vi "Lab Panel V5.24.2.vi"() -> ()   [LabVIEW 2013] (continued)
                          frame False {
                          }
                          frame True {
                            n2517 = Bundle(cluster=w4678, "amps"=w4682, "volts"=w4681, "pf"=w4680) -> (w4679:cluster{"amps":dbl, "volts":dbl, "pf":dbl})
                            n2518 = local write "ON L05-2"(w4679) -> ()
                          }
                        }
                      }
                      frame #1 {
                        n2519 = Unbundle(w4687) -> ("amps"=w4686:dbl, "volts"=w4685:dbl, "pf"=w4684:dbl)
                        n2520 = case shown="True" w4688 {
                          tunnel: w4695 -> [_ w4727]
                          tunnel: w4694 -> [_ w4734]
                          tunnel: w4693 -> [_ _]
                          tunnel: w4692 -> [_ _]
                          tunnel: w4691 -> [_ w4733]
                          tunnel: w4690 -> [_ w4732]
                          tunnel: w4689 -> [_ w4697]
                          tunnel: w4686 -> [_ w4729]
                          tunnel: w4685 -> [_ w4728]
                          tunnel: w4684 -> [_ w4726]
                          tunnel: w4683 -> [_ w4718]
                          frame False {
                          }
                          frame True {
                            n2521 = local read "TDMS LAB05-2"() -> (w4731:refnum<k34>)
                            n2522 = Build Array(w4728) -> (w4723:dbl[])
                            n2523 = Build Array(w4726) -> (w4722:dbl[])
                            n2524 = Build Array(w4733) -> (w4721:dbl[])
                            n2525 = Build Array(w4734) -> (w4720:dbl[])
                            n2526 = Build Array(w4729) -> (w4725:dbl[])
                            n2527 = Build Array(w4727) -> (w4724:dbl[])
                            n2528 = Build Array(w4732) -> (w4719:dbl[])
                            n2529 = Build Array("AMPS ON", "AMPS OFF", "VOLTS", "PF", "TEMP Live", "TEMP Neut", "CYCLE") -> (w4702:string[])
                            n2530 = Bundle By Name("Y"=w4725, "t0"=w4718) -> (w4717:waveform(dbl))  [unwired: 1 in]
                            n2531 = Bundle By Name("Y"=w4724, "t0"=w4718) -> (w4716:waveform(dbl))  [unwired: 1 in]
                            n2532 = Bundle By Name("Y"=w4723, "t0"=w4718) -> (w4715:waveform(dbl))  [unwired: 1 in]
                            n2533 = Bundle By Name("Y"=w4722, "t0"=w4718) -> (w4714:waveform(dbl))  [unwired: 1 in]
                            n2534 = Bundle By Name("Y"=w4721, "t0"=w4718) -> (w4713:waveform(dbl))  [unwired: 1 in]
                            n2535 = Bundle By Name("Y"=w4720, "t0"=w4718) -> (w4712:waveform(dbl))  [unwired: 1 in]
                            n2536 = Bundle By Name("Y"=w4719, "t0"=w4718) -> (w4711:waveform(dbl))  [unwired: 1 in]
                            n2537 = Build Array(w4717, w4716, w4715, w4714, w4713, w4712, w4711) -> (w4710:waveform(dbl)[])
                            n2538 = TDMS Write(0:w4731, 5:"TEST VALUES", 7:w4702, 9:w4710) -> (4:w4701:refnum<k34>, 6:w4700:string, 15:w4699:errorcluster)  [unwired: 2 in, 1 out]
                            n2539 = TDMS Write(0:w4701, 5:w4700, 7:"TIME", 9:w4697, 11:w4699) -> (15:w4696:errorcluster)  [unwired: 1 in, 3 out]
                            n2540 = local write "data file error"(w4696) -> ()
                          }
                        }
                      }
                    }
                  }
                }
              }
            }
          }
          frame #14 {
            # "display test values on chart"
            n2541 = local read "jig cycle"() -> (w4739:dbl)
            n2542 = local read "on loops"() -> (w4741:dbl)
            n2543 = Add(x=w4741, y=2) -> (x+y=w4738:dbl)
            n2544 = Equal?(x=w4739, y=1) -> (x = y?=w4737:bool)
            n2545 = Equal?(x=w4739, y=w4738) -> (x = y?=w4736:bool)
            n2546 = Or(x=w4737, y=w4736) -> (x .or. y?=w4735:bool)
            "graph flag" <- w4735
            n2547 = global write "Global display 3.vi" "graph flag"(w4735) -> ()
            n2548 = case shown="True" w4735 {
              frame False {
              }
              frame True {
                n2549 = local read "SIG LAB05-1"() -> (w4784:T2)
                n2550 = local read "SIG LAB04-2"() -> (w4785:T2)
                n2551 = local read "SIG LAB05-2"() -> (w4783:T2)
                n2552 = local read "SIG LAB04-1"() -> (w4786:T2)
                n2553 = local read "SIG LAB03-1"() -> (w4788:T2)
                n2554 = local read "SIG LAB03-2"() -> (w4787:T2)
                n2555 = local read "SIG LAB01-1"() -> (w4792:T2)
                n2556 = local read "SIG LAB02-2"() -> (w4789:T2)
                n2557 = local read "SIG LAB02-1"() -> (w4790:T2)
                n2558 = local read "SIG LAB01-2"() -> (w4791:T2)
                n2559 = Unbundle(w4785) -> ("AMPS"=w4775:dbl, "VOLTS"=w4765:dbl, "Tmp Live"=w4755:dbl, "Tmp Neut"=w4745:dbl)  [unwired: 1 out]
                n2560 = Unbundle(w4784) -> ("AMPS"=w4774:dbl, "VOLTS"=w4764:dbl, "Tmp Live"=w4754:dbl, "Tmp Neut"=w4744:dbl)  [unwired: 1 out]
                n2561 = Unbundle(w4783) -> ("AMPS"=w4773:dbl, "VOLTS"=w4763:dbl, "Tmp Live"=w4753:dbl, "Tmp Neut"=w4743:dbl)  [unwired: 1 out]
                n2562 = Unbundle(w4786) -> ("AMPS"=w4776:dbl, "VOLTS"=w4766:dbl, "Tmp Live"=w4756:dbl, "Tmp Neut"=w4746:dbl)  [unwired: 1 out]
                n2563 = Unbundle(w4787) -> ("AMPS"=w4777:dbl, "VOLTS"=w4767:dbl, "Tmp Live"=w4757:dbl, "Tmp Neut"=w4747:dbl)  [unwired: 1 out]
                n2564 = Unbundle(w4788) -> ("AMPS"=w4778:dbl, "VOLTS"=w4768:dbl, "Tmp Live"=w4758:dbl, "Tmp Neut"=w4748:dbl)  [unwired: 1 out]
                n2565 = Unbundle(w4789) -> ("AMPS"=w4779:dbl, "VOLTS"=w4769:dbl, "Tmp Live"=w4759:dbl, "Tmp Neut"=w4749:dbl)  [unwired: 1 out]
                n2566 = Unbundle(w4790) -> ("AMPS"=w4780:dbl, "VOLTS"=w4770:dbl, "Tmp Live"=w4760:dbl, "Tmp Neut"=w4750:dbl)  [unwired: 1 out]
                n2567 = Unbundle(w4792) -> ("AMPS"=w4782:dbl, "VOLTS"=w4772:dbl, "Tmp Live"=w4762:dbl, "Tmp Neut"=w4752:dbl)  [unwired: 1 out]
                n2568 = Unbundle(w4791) -> ("AMPS"=w4781:dbl, "VOLTS"=w4771:dbl, "Tmp Live"=w4761:dbl, "Tmp Neut"=w4751:dbl)  [unwired: 1 out]
                n2569 = stacked-sequence {
                  tunnel: w4782 -> [w4824 _ _]
                  tunnel: w4781 -> [w4823 _ _]
                  tunnel: w4780 -> [w4814 _ _]
                  tunnel: w4779 -> [w4813 _ _]
                  tunnel: w4778 -> [w4803 _ _]
                  tunnel: w4777 -> [w4802 _ _]
                  tunnel: w4776 -> [_ w4847 _]
                  tunnel: w4775 -> [_ w4846 _]
                  tunnel: w4774 -> [_ w4836 _]
                  tunnel: w4773 -> [_ w4835 _]
                  tunnel: w4772 -> [w4821 _ _]
                  tunnel: w4771 -> [w4820 _ _]
                  tunnel: w4770 -> [w4811 _ _]
                  tunnel: w4769 -> [w4810 _ _]
                  tunnel: w4768 -> [w4801 _ _]
                  tunnel: w4767 -> [w4800 _ _]
                  tunnel: w4766 -> [_ w4845 _]
                  tunnel: w4765 -> [_ w4844 _]
                  tunnel: w4764 -> [_ w4834 _]
                  tunnel: w4763 -> [_ w4833 _]
                  tunnel: w4762 -> [w4818 _ _]
                  tunnel: w4761 -> [w4816 _ _]
                  tunnel: w4760 -> [w4807 _ _]
                  tunnel: w4759 -> [w4805 _ _]
                  tunnel: w4758 -> [w4799 _ _]
                  tunnel: w4757 -> [w4797 _ _]
                  tunnel: w4756 -> [_ w4843 _]
                  tunnel: w4755 -> [_ w4841 _]
                  tunnel: w4754 -> [_ w4832 _]
                  tunnel: w4753 -> [_ w4830 _]
                  tunnel: w4752 -> [w4817 _ _]
                  tunnel: w4751 -> [w4815 _ _]
                  tunnel: w4750 -> [w4806 _ _]
                  tunnel: w4749 -> [w4804 _ _]
                  tunnel: w4748 -> [w4798 _ _]
                  tunnel: w4747 -> [w4796 _ _]
                  tunnel: w4746 -> [_ w4842 _]
                  tunnel: w4745 -> [_ w4840 _]
                  tunnel: w4744 -> [_ w4831 _]
                  tunnel: w4743 -> [_ w4829 _]
                  frame #0 {
                    n2570 = Merge Signals(w4824, w4823) -> (→"LAB01 AMPS":dynamicdata)
                    n2571 = Merge Signals(w4821, w4820) -> (→"LAB01 VOLTS":dynamicdata)
                    n2572 = Merge Signals(w4801, w4800) -> (→"LAB03 VOLTS":dynamicdata)
                    n2573 = Merge Signals(w4818, w4817, w4816, w4815) -> (→"LAB01 deg C":dynamicdata)
                    n2574 = Merge Signals(w4814, w4813) -> (→"LAB02 AMPS":dynamicdata)
                    n2575 = Merge Signals(w4807, w4806, w4805, w4804) -> (→"LAB02 deg C":dynamicdata)
                    n2576 = Merge Signals(w4799, w4798, w4797, w4796) -> (→"LAB03 deg C":dynamicdata)
                    n2577 = Merge Signals(w4811, w4810) -> (→"LAB02 VOLTS":dynamicdata)
                    n2578 = Merge Signals(w4803, w4802) -> (→"LAB03 AMPS":dynamicdata)
                  }
                  frame #1 {
                    n2579 = Merge Signals(w4834, w4833) -> (→"LAB05 VOLTS":dynamicdata)
                    n2580 = Merge Signals(w4847, w4846) -> (→"LAB04 AMPS":dynamicdata)
                    n2581 = Merge Signals(w4836, w4835) -> (→"LAB05 AMPS":dynamicdata)
                    n2582 = Merge Signals(w4832, w4831, w4830, w4829) -> (→"LAB05 deg C":dynamicdata)
                    n2583 = Merge Signals(w4843, w4842, w4841, w4840) -> (→"LAB04 deg C":dynamicdata)
                    n2584 = Merge Signals(w4845, w4844) -> (→"LAB04 VOLTS":dynamicdata)
                  }
                  frame #2 {
                    n2585 = local read "LAB05 VOLTS"() -> (w4855:dynamicdata)
                    n2586 = local read "LAB04 VOLTS"() -> (w4856:dynamicdata)
                    n2587 = local read "LAB02 VOLTS"() -> (w4858:dynamicdata)
                    n2588 = local read "LAB03 VOLTS"() -> (w4857:dynamicdata)
                    n2589 = local read "LAB05 AMPS"() -> (w4861:dynamicdata)
                    n2590 = local read "LAB01 VOLTS"() -> (w4859:dynamicdata)
                    n2591 = local read "LAB04 AMPS"() -> (w4862:dynamicdata)
                    n2592 = local read "LAB03 AMPS"() -> (w4863:dynamicdata)
                    n2593 = local read "LAB03 deg C"() -> (w4851:dynamicdata)
                    n2594 = local read "LAB02 AMPS"() -> (w4864:dynamicdata)
                    n2595 = local read "LAB04 deg C"() -> (w4850:dynamicdata)
                    n2596 = local read "LAB05 deg C"() -> (w4849:dynamicdata)
                    n2597 = local read "LAB02 deg C"() -> (w4852:dynamicdata)
                    n2598 = local read "LAB01 deg C"() -> (w4853:dynamicdata)
                    n2599 = local read "LAB01 AMPS"() -> (w4865:dynamicdata)
                    n2600 = Merge Signals(w4853, w4852, w4851, w4850, w4849) -> (w4848:dynamicdata)
                    n2601 = Merge Signals(w4865, w4864, w4863, w4862, w4861) -> (w4860:dynamicdata)
                    n2602 = Merge Signals(w4859, w4858, w4857, w4856, w4855) -> (w4854:dynamicdata)
                    n2603 = global write "Global display 3.vi" "graph volts"(w4854) -> ()
                    n2604 = global write "Global display 3.vi" "graph deg C"(w4848) -> ()
                    n2605 = global write "Global display 3.vi" "graph amps"(w4860) -> ()
                  }
                }
              }
            }
          }
          frame #15 {
            # "check for amps fail"
            # "check for cycle test & temperature rise fail conditions"
            n2606 = local read "on loops"() -> (w4892:dbl)
            n2607 = local read "jig cycle"() -> (w4889:dbl)
            n2608 = local read "jig cycle"() -> (w4894:dbl)
            n2609 = Add(x=w4892, y=3.0) -> (x+y=w4890:dbl)
            n2610 = Equal?(x=w4889, y=w4890) -> (x = y?=w4885:bool)
            n2611 = local read "Fail Loops"() -> (w4866:dbl)
            n2612 = Equal?(x=w4894, y=1.0) -> (x = y?=w4887:bool)
            n2613 = global write "Global 1.vi" "fail count"(w4866) -> ()
            n2614 = stacked-sequence {
              tunnel: w4888 -> [w4897 _ _ _ _ _ _ _ _ _]
              tunnel: w4887 -> [w4898 w4918 w4938 w4958 w4978 w4998 w5018 w5038 w5058 w5078]
              tunnel: w4886 -> [w4895 _ _ _ _ _ _ _ _ _]
              tunnel: w4885 -> [w4896 w4917 w4937 w4957 w4977 w4997 w5017 w5037 w5057 w5077]
              tunnel: w4884 -> [_ w4916 _ _ _ _ _ _ _ _]
              tunnel: w4883 -> [_ w4915 _ _ _ _ _ _ _ _]
              tunnel: w4882 -> [_ _ w4936 _ _ _ _ _ _ _]
              tunnel: w4881 -> [_ _ w4935 _ _ _ _ _ _ _]
              tunnel: w4880 -> [_ _ _ w4956 _ _ _ _ _ _]
              tunnel: w4879 -> [_ _ _ w4955 _ _ _ _ _ _]
              tunnel: w4878 -> [_ _ _ _ w4976 _ _ _ _ _]
              tunnel: w4877 -> [_ _ _ _ w4975 _ _ _ _ _]
              tunnel: w4876 -> [_ _ _ _ _ w4996 _ _ _ _]
              tunnel: w4875 -> [_ _ _ _ _ w4995 _ _ _ _]
              tunnel: w4874 -> [_ _ _ _ _ _ w5016 _ _ _]
              tunnel: w4873 -> [_ _ _ _ _ _ w5015 _ _ _]
              tunnel: w4872 -> [_ _ _ _ _ _ _ w5036 _ _]
              tunnel: w4871 -> [_ _ _ _ _ _ _ w5035 _ _]
              tunnel: w4870 -> [_ _ _ _ _ _ _ _ w5056 _]
              tunnel: w4869 -> [_ _ _ _ _ _ _ _ w5055 _]
              tunnel: w4868 -> [_ _ _ _ _ _ _ _ _ w5076]
              tunnel: w4867 -> [_ _ _ _ _ _ _ _ _ w5075]
              frame #0 {
                # "LAB01-1"
                n2615 = case shown="True" w4895 {
                  tunnel: w4898 -> [_ w4911]
                  tunnel: w4897 -> [_ w4908]
                  tunnel: w4896 -> [_ w4907]
                  frame False {
                  }
                  frame True {
                    n2616 = local read "TEMP START LAB01-1"() -> (w4913:cluster{"TL":dbl, "TN":dbl})
                    n2617 = local read "RESULT LAB01-1"() -> (w4902:bool)
                    n2618 = local read "FAIL LAB01-1"() -> (w4905:cluster{"LO":dbl, "HI":dbl})
                    n2619 = local read "TDMS LAB01-1"() -> (w4912:refnum<k34>)
                    n2620 = local read "SET LAB01-1"() -> (w4909:T5)
                    n2621 = local read "DISP LAB01-1"() -> (w4910:T4)
                    n2622 = local read "SIG LAB01-1"() -> (w4914:T2)
                    n2623 = Bundle("FAIL LAB01-1"=w4905, "SIG LAB01-1"=w4914, "TEMP START LAB01-1"=w4913, "DISP LAB01-1"=w4910, "SET LAB01-1"=w4909, "TDMS LAB01-1"=w4912) -> (w4899:T33)  [unwired: 1 in]
                    n2624 = call "sub vi - cycle&temp fail v7.vi"("Amps Lo?"=w4911, "Input Cluster"=w4899, "SELECT"=w4908, "Amps Hi?"=w4907, "Result In"=w4902) -> ("(FAIL) out"=w4904:cluster{"FAIL LO":dbl, "FAIL HI":dbl}, "(DISP) out"=w4900:T4, "T-RISE"=w4901:cluster{"T-RISE (L)":dbl, "T-RISE (N)":dbl}, "Result Out"=w4903:bool, "file error"=w4906:errorcluster)  [unwired: 10 in]
                    n2625 = local write "TEMP RISE LAB01-1"(w4901) -> ()
                    n2626 = local write "FAIL LAB01-1"(w4904) -> ()
                    n2627 = local write "DISP LAB01-1"(w4900) -> ()
                    n2628 = local write "RESULT LAB01-1"(w4903) -> ()
                    n2629 = local write "data file error"(w4906) -> ()
                  }
                }
              }
              frame #1 {
                # "LAB01-2"
                n2630 = case shown="True" w4916 {
                  tunnel: w4918 -> [_ w4931]
                  tunnel: w4915 -> [_ w4928]
                  tunnel: w4917 -> [_ w4927]
                  frame False {
                  }
                  frame True {
                    n2631 = local read "TEMP START LAB01-2"() -> (w4933:cluster{"TL":dbl, "TN":dbl})
                    n2632 = local read "FAIL LAB01-2"() -> (w4924:cluster{"LO":dbl, "HI":dbl})
                    n2633 = local read "TDMS LAB01-2"() -> (w4932:refnum<k34>)
                    n2634 = local read "SET LAB01-2"() -> (w4929:T5)
                    n2635 = local read "DISP LAB01-2"() -> (w4930:T4)
                    n2636 = local read "RESULT LAB01-2"() -> (w4921:bool)
                    n2637 = local read "SIG LAB01-2"() -> (w4934:T2)
                    n2638 = Bundle("FAIL LAB01-2"=w4924, "SIG LAB01-2"=w4934, "TEMP START LAB01-2"=w4933, "DISP LAB01-2"=w4930, "SET LAB01-2"=w4929, "TDMS LAB01-2"=w4932) -> (w4919:T34)  [unwired: 1 in]
                    n2639 = call "sub vi - cycle&temp fail v7.vi"("Amps Lo?"=w4931, "Input Cluster"=w4919, "SELECT"=w4928, "Amps Hi?"=w4927, "Result In"=w4921) -> ("(FAIL) out"=w4923:cluster{"FAIL LO":dbl, "FAIL HI":dbl}, "(DISP) out"=w4926:T4, "T-RISE"=w4920:cluster{"T-RISE (L)":dbl, "T-RISE (N)":dbl}, "Result Out"=w4922:bool, "file error"=w4925:errorcluster)  [unwired: 10 in]
                    n2640 = local write "TEMP RISE LAB01-2"(w4920) -> ()
                    n2641 = local write "FAIL LAB01-2"(w4923) -> ()
                    n2642 = local write "DISP LAB01-2"(w4926) -> ()
                    n2643 = local write "RESULT LAB01-2"(w4922) -> ()
                    n2644 = local write "data file error"(w4925) -> ()
                  }
                }
              }
              frame #2 {
                # "LAB02-1"
                n2645 = case shown="True" w4936 {
                  tunnel: w4938 -> [_ w4951]
                  tunnel: w4935 -> [_ w4948]
                  tunnel: w4937 -> [_ w4947]
                  frame False {
                  }
                  frame True {
                    n2646 = local read "TEMP START LAB02-1"() -> (w4953:cluster{"TL":dbl, "TN":dbl})
                    n2647 = local read "FAIL LAB02-1"() -> (w4944:cluster{"LO":dbl, "HI":dbl})
                    n2648 = local read "TDMS LAB02-1"() -> (w4952:refnum<k34>)
                    n2649 = local read "SET LAB02-1"() -> (w4949:T5)
                    n2650 = local read "DISP LAB02-1"() -> (w4950:T4)
                    n2651 = local read "SIG LAB02-1"() -> (w4954:T2)
                    n2652 = local read "RESULT LAB02-1"() -> (w4941:bool)
                    n2653 = Bundle("FAIL LAB02-1"=w4944, "SIG LAB02-1"=w4954, "TEMP START LAB02-1"=w4953, "DISP LAB02-1"=w4950, "SET LAB02-1"=w4949, "TDMS LAB02-1"=w4952) -> (w4939:T35)  [unwired: 1 in]
                    n2654 = call "sub vi - cycle&temp fail v7.vi"("Amps Lo?"=w4951, "Input Cluster"=w4939, "SELECT"=w4948, "Amps Hi?"=w4947, "Result In"=w4941) -> ("(FAIL) out"=w4943:cluster{"FAIL LO":dbl, "FAIL HI":dbl}, "(DISP) out"=w4946:T4, "T-RISE"=w4940:cluster{"T-RISE (L)":dbl, "T-RISE (N)":dbl}, "Result Out"=w4942:bool, "file error"=w4945:errorcluster)  [unwired: 10 in]
                    n2655 = local write "TEMP RISE LAB02-1"(w4940) -> ()
                    n2656 = local write "FAIL LAB02-1"(w4943) -> ()
                    n2657 = local write "DISP LAB02-1"(w4946) -> ()
                    n2658 = local write "RESULT LAB02-1"(w4942) -> ()
                    n2659 = local write "data file error"(w4945) -> ()
                  }
                }
              }
              frame #3 {
                # "LAB02-2"
                n2660 = case shown="True" w4956 {
                  tunnel: w4958 -> [_ w4971]
                  tunnel: w4955 -> [_ w4968]
                  tunnel: w4957 -> [_ w4967]
                  frame False {
                  }
                  frame True {
                    n2661 = local read "TEMP START LAB02-2"() -> (w4973:cluster{"TL":dbl, "TN":dbl})
                    n2662 = local read "FAIL LAB02-2"() -> (w4964:cluster{"LO":dbl, "HI":dbl})
                    n2663 = local read "TDMS LAB02-2"() -> (w4972:refnum<k34>)
                    n2664 = local read "SET LAB02-2"() -> (w4969:T5)
                    n2665 = local read "DISP LAB02-2"() -> (w4970:T4)
                    n2666 = local read "SIG LAB02-2"() -> (w4974:T2)
                    n2667 = local read "RESULT LAB02-2"() -> (w4961:bool)
                    n2668 = Bundle("FAIL LAB02-2"=w4964, "SIG LAB02-2"=w4974, "TEMP START LAB02-2"=w4973, "DISP LAB02-2"=w4970, "SET LAB02-2"=w4969, "TDMS LAB02-2"=w4972) -> (w4959:T36)  [unwired: 1 in]
                    n2669 = call "sub vi - cycle&temp fail v7.vi"("Amps Lo?"=w4971, "Input Cluster"=w4959, "SELECT"=w4968, "Amps Hi?"=w4967, "Result In"=w4961) -> ("(FAIL) out"=w4963:cluster{"FAIL LO":dbl, "FAIL HI":dbl}, "(DISP) out"=w4966:T4, "T-RISE"=w4960:cluster{"T-RISE (L)":dbl, "T-RISE (N)":dbl}, "Result Out"=w4962:bool, "file error"=w4965:errorcluster)  [unwired: 10 in]
                    n2670 = local write "TEMP RISE LAB02-2"(w4960) -> ()
                    n2671 = local write "FAIL LAB02-2"(w4963) -> ()
                    n2672 = local write "DISP LAB02-2"(w4966) -> ()
                    n2673 = local write "RESULT LAB02-2"(w4962) -> ()
                    n2674 = local write "data file error"(w4965) -> ()
                  }
                }
              }
              frame #4 {
                # "LAB03-1"
                n2675 = case shown="True" w4976 {
                  tunnel: w4978 -> [_ w4991]
                  tunnel: w4975 -> [_ w4988]
                  tunnel: w4977 -> [_ w4987]
                  frame False {
                  }
                  frame True {
                    n2676 = local read "TEMP START LAB03-1"() -> (w4993:cluster{"TL":dbl, "TN":dbl})
                    n2677 = local read "FAIL LAB03-1"() -> (w4984:cluster{"LO":dbl, "HI":dbl})
                    n2678 = local read "TDMS LAB03-1"() -> (w4992:refnum<k34>)
                    n2679 = local read "SET LAB03-1"() -> (w4989:T5)
                    n2680 = local read "DISP LAB03-1"() -> (w4990:T4)
                    n2681 = local read "SIG LAB03-1"() -> (w4994:T2)
                    n2682 = local read "RESULT LAB03-1"() -> (w4981:bool)
                    n2683 = Bundle("FAIL LAB03-1"=w4984, "SIG LAB03-1"=w4994, "TEMP START LAB03-1"=w4993, "DISP LAB03-1"=w4990, "SET LAB03-1"=w4989, "TDMS LAB03-1"=w4992) -> (w4979:T37)  [unwired: 1 in]
                    n2684 = call "sub vi - cycle&temp fail v7.vi"("Amps Lo?"=w4991, "Input Cluster"=w4979, "SELECT"=w4988, "Amps Hi?"=w4987, "Result In"=w4981) -> ("(FAIL) out"=w4983:cluster{"FAIL LO":dbl, "FAIL HI":dbl}, "(DISP) out"=w4986:T4, "T-RISE"=w4980:cluster{"T-RISE (L)":dbl, "T-RISE (N)":dbl}, "Result Out"=w4982:bool, "file error"=w4985:errorcluster)  [unwired: 10 in]
                    n2685 = local write "TEMP RISE LAB03-1"(w4980) -> ()
                    n2686 = local write "FAIL LAB03-1"(w4983) -> ()
                    n2687 = local write "DISP LAB03-1"(w4986) -> ()
                    n2688 = local write "RESULT LAB03-1"(w4982) -> ()
                    n2689 = local write "data file error"(w4985) -> ()
                  }
                }
              }
              frame #5 {
                # "LAB03-2"
                n2690 = case shown="True" w4996 {
                  tunnel: w4998 -> [_ w5011]
                  tunnel: w4995 -> [_ w5008]
                  tunnel: w4997 -> [_ w5007]
                  frame False {
                  }
                  frame True {
                    n2691 = local read "TEMP START LAB03-2"() -> (w5013:cluster{"TL":dbl, "TN":dbl})
                    n2692 = local read "FAIL LAB03-2"() -> (w5004:cluster{"LO":dbl, "HI":dbl})
                    n2693 = local read "TDMS LAB03-2"() -> (w5012:refnum<k34>)
                    n2694 = local read "SET LAB03-2"() -> (w5009:T5)
                    n2695 = local read "DISP LAB03-2"() -> (w5010:T4)
                    n2696 = local read "RESULT LAB03-2"() -> (w5001:bool)
                    n2697 = local read "SIG LAB03-2"() -> (w5014:T2)
                    n2698 = Bundle("FAIL LAB03-2"=w5004, "SIG LAB03-2"=w5014, "TEMP START LAB03-2"=w5013, "DISP LAB03-2"=w5010, "SET LAB03-2"=w5009, "TDMS LAB03-2"=w5012) -> (w4999:T38)  [unwired: 1 in]
                    n2699 = call "sub vi - cycle&temp fail v7.vi"("Amps Lo?"=w5011, "Input Cluster"=w4999, "SELECT"=w5008, "Amps Hi?"=w5007, "Result In"=w5001) -> ("(FAIL) out"=w5003:cluster{"FAIL LO":dbl, "FAIL HI":dbl}, "(DISP) out"=w5006:T4, "T-RISE"=w5000:cluster{"T-RISE (L)":dbl, "T-RISE (N)":dbl}, "Result Out"=w5002:bool, "file error"=w5005:errorcluster)  [unwired: 10 in]
                    n2700 = local write "FAIL LAB03-2"(w5003) -> ()
                    n2701 = local write "TEMP RISE LAB03-2"(w5000) -> ()
                    n2702 = local write "DISP LAB03-2"(w5006) -> ()
                    n2703 = local write "RESULT LAB03-2"(w5002) -> ()
                    n2704 = local write "data file error"(w5005) -> ()
                  }
                }
              }
              frame #6 {
                # "LAB04-1"
                n2705 = case shown="True" w5016 {
                  tunnel: w5018 -> [_ w5031]
                  tunnel: w5015 -> [_ w5028]
                  tunnel: w5017 -> [_ w5027]
                  frame False {
                  }
                  frame True {
                    n2706 = local read "TEMP START LAB04-1"() -> (w5033:cluster{"TL":dbl, "TN":dbl})
                    n2707 = local read "FAIL LAB04-1"() -> (w5024:cluster{"LO":dbl, "HI":dbl})
                    n2708 = local read "TDMS LAB04-1"() -> (w5032:refnum<k34>)
                    n2709 = local read "SET LAB04-1"() -> (w5029:T5)
                    n2710 = local read "DISP LAB04-1"() -> (w5030:T4)
                    n2711 = local read "SIG LAB04-1"() -> (w5034:T2)
                    n2712 = local read "RESULT LAB04-1"() -> (w5021:bool)
                    n2713 = Bundle("FAIL LAB04-1"=w5024, "SIG LAB04-1"=w5034, "TEMP START LAB04-1"=w5033, "DISP LAB04-1"=w5030, "SET LAB04-1"=w5029, "TDMS LAB04-1"=w5032) -> (w5019:T39)  [unwired: 1 in]
                    n2714 = call "sub vi - cycle&temp fail v7.vi"("Amps Lo?"=w5031, "Input Cluster"=w5019, "SELECT"=w5028, "Amps Hi?"=w5027, "Result In"=w5021) -> ("(FAIL) out"=w5023:cluster{"FAIL LO":dbl, "FAIL HI":dbl}, "(DISP) out"=w5026:T4, "T-RISE"=w5020:cluster{"T-RISE (L)":dbl, "T-RISE (N)":dbl}, "Result Out"=w5022:bool, "file error"=w5025:errorcluster)  [unwired: 10 in]
                    n2715 = local write "TEMP RISE LAB04-1"(w5020) -> ()
                    n2716 = local write "FAIL LAB04-1"(w5023) -> ()
                    n2717 = local write "DISP LAB04-1"(w5026) -> ()
                    n2718 = local write "RESULT LAB04-1"(w5022) -> ()
                    n2719 = local write "data file error"(w5025) -> ()
                  }
                }
              }
              frame #7 {
                # "LAB04-2"
                n2720 = case shown="True" w5036 {
                  tunnel: w5038 -> [_ w5051]
                  tunnel: w5035 -> [_ w5048]
                  tunnel: w5037 -> [_ w5047]
                  frame False {
                  }
                  frame True {
                    n2721 = local read "TEMP START LAB04-2"() -> (w5053:cluster{"TL":dbl, "TN":dbl})
                    n2722 = local read "FAIL LAB04-2"() -> (w5044:cluster{"LO":dbl, "HI":dbl})
                    n2723 = local read "TDMS LAB04-2"() -> (w5052:refnum<k34>)
                    n2724 = local read "SET LAB04-2"() -> (w5049:T5)
                    n2725 = local read "DISP LAB04-2"() -> (w5050:T4)
                    n2726 = local read "SIG LAB04-2"() -> (w5054:T2)
                    n2727 = local read "RESULT LAB04-2"() -> (w5041:bool)
                    n2728 = Bundle("FAIL LAB04-2"=w5044, "SIG LAB04-2"=w5054, "TEMP START LAB04-2"=w5053, "DISP LAB04-2"=w5050, "SET LAB04-2"=w5049, "TDMS LAB04-2"=w5052) -> (w5039:T40)  [unwired: 1 in]
                    n2729 = call "sub vi - cycle&temp fail v7.vi"("Amps Lo?"=w5051, "Input Cluster"=w5039, "SELECT"=w5048, "Amps Hi?"=w5047, "Result In"=w5041) -> ("(FAIL) out"=w5043:cluster{"FAIL LO":dbl, "FAIL HI":dbl}, "(DISP) out"=w5046:T4, "T-RISE"=w5040:cluster{"T-RISE (L)":dbl, "T-RISE (N)":dbl}, "Result Out"=w5042:bool, "file error"=w5045:errorcluster)  [unwired: 10 in]
                    n2730 = local write "TEMP RISE LAB04-2"(w5040) -> ()
                    n2731 = local write "FAIL LAB04-2"(w5043) -> ()
                    n2732 = local write "DISP LAB04-2"(w5046) -> ()
                    n2733 = local write "RESULT LAB04-2"(w5042) -> ()
                    n2734 = local write "data file error"(w5045) -> ()
                  }
                }
              }
              frame #8 {
                # "LAB05-1"
                n2735 = case shown="True" w5056 {
                  tunnel: w5058 -> [_ w5071]
                  tunnel: w5055 -> [_ w5068]
                  tunnel: w5057 -> [_ w5067]
                  frame False {
                  }
                  frame True {
                    n2736 = local read "TEMP START LAB05-1"() -> (w5073:cluster{"TL":dbl, "TN":dbl})
                    n2737 = local read "FAIL LAB05-1"() -> (w5064:cluster{"LO":dbl, "HI":dbl})
                    n2738 = local read "TDMS LAB05-1"() -> (w5072:refnum<k34>)
                    n2739 = local read "SET LAB05-1"() -> (w5069:T5)
                    n2740 = local read "DISP LAB05-1"() -> (w5070:T4)
                    n2741 = local read "SIG LAB05-1"() -> (w5074:T2)
                    n2742 = local read "RESULT LAB05-1"() -> (w5061:bool)
                    n2743 = Bundle("FAIL LAB05-1"=w5064, "SIG LAB05-1"=w5074, "TEMP START LAB05-1"=w5073, "DISP LAB05-1"=w5070, "SET LAB05-1"=w5069, "TDMS LAB05-1"=w5072) -> (w5059:T41)  [unwired: 1 in]
                    n2744 = call "sub vi - cycle&temp fail v7.vi"("Amps Lo?"=w5071, "Input Cluster"=w5059, "SELECT"=w5068, "Amps Hi?"=w5067, "Result In"=w5061) -> ("(FAIL) out"=w5063:cluster{"FAIL LO":dbl, "FAIL HI":dbl}, "(DISP) out"=w5066:T4, "T-RISE"=w5060:cluster{"T-RISE (L)":dbl, "T-RISE (N)":dbl}, "Result Out"=w5062:bool, "file error"=w5065:errorcluster)  [unwired: 10 in]
                    n2745 = local write "TEMP RISE LAB05-1"(w5060) -> ()
                    n2746 = local write "FAIL LAB05-1"(w5063) -> ()
                    n2747 = local write "DISP LAB05-1"(w5066) -> ()
                    n2748 = local write "RESULT LAB05-1"(w5062) -> ()
                    n2749 = local write "data file error"(w5065) -> ()
                  }
                }
              }
              frame #9 {
                # "LAB05-2"
                n2750 = case shown="True" w5076 {
                  tunnel: w5078 -> [_ w5091]
                  tunnel: w5075 -> [_ w5088]
                  tunnel: w5077 -> [_ w5087]
                  frame False {
                  }
                  frame True {
                    n2751 = local read "TEMP START LAB05-2"() -> (w5093:cluster{"TL":dbl, "TN":dbl})
                    n2752 = local read "FAIL LAB05-2"() -> (w5084:cluster{"LO":dbl, "HI":dbl})
                    n2753 = local read "TDMS LAB05-2"() -> (w5092:refnum<k34>)
                    n2754 = local read "SET LAB05-2"() -> (w5089:T5)
                    n2755 = local read "DISP LAB05-2"() -> (w5090:T4)
                    n2756 = local read "SIG LAB05-2"() -> (w5094:T2)
                    n2757 = local read "RESULT LAB05-2"() -> (w5081:bool)
                    n2758 = Bundle("FAIL LAB05-2"=w5084, "SIG LAB05-2"=w5094, "TEMP START LAB05-2"=w5093, "DISP LAB05-2"=w5090, "SET LAB05-2"=w5089, "TDMS LAB05-2"=w5092) -> (w5079:T42)  [unwired: 1 in]
                    n2759 = call "sub vi - cycle&temp fail v7.vi"("Amps Lo?"=w5091, "Input Cluster"=w5079, "SELECT"=w5088, "Amps Hi?"=w5087, "Result In"=w5081) -> ("(FAIL) out"=w5083:cluster{"FAIL LO":dbl, "FAIL HI":dbl}, "(DISP) out"=w5086:T4, "T-RISE"=w5080:cluster{"T-RISE (L)":dbl, "T-RISE (N)":dbl}, "Result Out"=w5082:bool, "file error"=w5085:errorcluster)  [unwired: 10 in]
                    n2760 = local write "TEMP RISE LAB05-2"(w5080) -> ()
                    n2761 = local write "FAIL LAB05-2"(w5083) -> ()
                    n2762 = local write "DISP LAB05-2"(w5086) -> ()
                    n2763 = local write "RESULT LAB05-2"(w5082) -> ()
                    n2764 = local write "data file error"(w5085) -> ()
                  }
                }
              }
            }
          }
          frame #16 {
            # "run calibration routine"
            n2765 = local read "SET (cal)"() -> (w5095:bool)
            n2766 = case shown="True" w5095 {
              frame False {
              }
              frame True {
                n2767 = stacked-sequence {
                  seq-local: [w5096 _ _] -> [_ w5098 _]
                  frame #0 {
                    n2768 = call "CALIBRATION PASSWORD"() -> ("PASSWORD"=w5096:string)  [unwired: 17 in, 2 out]
                  }
                  frame #1 {
                    n2769 = Equal?(x=w5098, y="7777") -> (x = y?=w5097:bool)
                    n2770 = case shown="True" w5097 {
                      frame False {
                      }
                      frame True {
                        n2771 = stacked-sequence {
                          frame #0 {
                            n2772 = local read "Temp Test Cal"() -> (w5100:dbl)
                            n2773 = call "sub vi - calibration v1.vi"("Temp Test Cal"=w5100) -> ()  [unwired: 11 in]
                          }
                          frame #1 {
                            n2774 = call "sub vi - get calibration values v1.vi"() -> ("TEMP REF CAL"=w5101:dbl, "LAB01 (CAL)"=w5106:T14, "LAB02 (CAL)"=w5105:T15, "LAB03 (CAL)"=w5104:T14, "LAB04 (CAL)"=w5103:T14, "calibration file error out"=w5107:errorcluster, "LAB05 (CAL)"=w5102:T14)  [unwired: 9 in]
                            n2775 = local write "TEMP REF cal"(w5101) -> ()
                            n2776 = local write "cal file error out"(w5107) -> ()
                            n2777 = local write "CAL LAB04"(w5103) -> ()
                            n2778 = local write "CAL LAB05"(w5102) -> ()
                            n2779 = local write "CAL LAB01"(w5106) -> ()
                            n2780 = local write "CAL LAB02"(w5105) -> ()
                            n2781 = local write "CAL LAB03"(w5104) -> ()
                          }
                        }
                      }
                    }
                  }
                  frame #2 {
                    n2782 = local write "SET (cal)"(FALSE) -> ()
                  }
                }
              }
            }
          }
          frame #17 {
            # "save certain settings to file"
            n2783 = String To Path(string="c:\\crabtree\\Set Up\\") -> (path=w5110:path)
            n2784 = Build Path(base path=w5110, name or relative path="settings.bin") -> (appended path=w5112:path)
            n2785 = Build Path(base path=w5110, name or relative path="mail.bin") -> (appended path=w5109:path)
            n2786 = Create Folder(path (use dialog)=w5110) -> (error out=w5115:errorcluster)  [unwired: 2 in, 2 out]
            n2787 = call <vilib>:"Clear Errors.vi"("error in (no error)"=w5115) -> ()  [unwired: 6 in, 1 out]
            n2788 = stacked-sequence {
              seq-local: [w5127 _] -> [_ w5140]
              tunnel: w5112 -> [_ w5141]
              tunnel: w5109 -> [_ w5139]
              frame #0 {
                n2789 = local read "C drive data root dir"() -> (w5126:path)
                n2790 = local read "Select COM port"() -> (w5123:refnum<visa-resource-name>)
                n2791 = local read "Network Directory"() -> (w5132:path)
                n2792 = local read "SET LAB05-2"() -> (w5131:T5)
                n2793 = local read "SET LAB05-1"() -> (w5130:T5)
                n2794 = local read "SET LAB04-2"() -> (w5129:T5)
                n2795 = local read "SET LAB03-2"() -> (w5133:T5)
                n2796 = local read "SET LAB04-1"() -> (w5128:T5)
                n2797 = local read "SET LAB03-1"() -> (w5134:T5)
                n2798 = local read "SET LAB02-2"() -> (w5135:T5)
                n2799 = local read "SET LAB02-1"() -> (w5136:T5)
                n2800 = local read "Temp Delay Lps"() -> (w5122:dbl)
                n2801 = local read "Amps Fail level"() -> (w5118:dbl)
                n2802 = local read "SET LAB01-2"() -> (w5137:T5)
                n2803 = local read "Temp Test Cal"() -> (w5119:dbl)
                n2804 = local read "SET LAB01-1"() -> (w5138:T5)
                n2805 = local read "Mail Test File To:"() -> (w5117:string)
                n2806 = local read "Temp Value"() -> (w5121:dbl)
                n2807 = local read "Fail Loops"() -> (w5120:dbl)
                n2808 = local read "Mail Test Fail"() -> (w5116:bool)
                n2809 = local read "RATE (Hz)"() -> (w5125:dbl)
                n2810 = local read "SAMPLES"() -> (w5124:dbl)
                n2811 = Bundle("SET LAB01-1"=w5138, "SET LAB01-2"=w5137, "SET LAB02-1"=w5136, "SET LAB02-2"=w5135, "SET LAB03-1"=w5134, "SET LAB03-2"=w5133, "SET LAB04-1"=w5128, "SET LAB04-2"=w5129, "SET LAB05-1"=w5130, "SET LAB05-2"=w5131, "Network Directory"=w5132, "C drive data root dir"=w5126, "RATE (Hz)"=w5125, "SAMPLES"=w5124, "Select COM port"=w5123, "Temp Delay Lps"=w5122, "Temp Value"=w5121, "Fail Loops"=w5120, "Temp Test Cal"=w5119, "Amps Fail level"=w5118, "Mail Test File To:"=w5117, "Mail Test Fail"=w5116) -> (w5127:T22)  [unwired: 1 in]
              }
              frame #1 {
                n2812 = event shown="[1] \"SET LAB01-1\", \"SET LAB01-2\", \"SET LAB02-1\", \"SET LAB02-2\", \"SET LAB03-1\", \"SET LAB03-2\", \"SET LAB04-1\", \"SET LAB04-2\", \"SET LAB05-1\", \"SET LAB05-2\", \"Network Directory\", \"C drive data root dir\", \"RATE (Hz)\", \"SAMPLES\", \"Select COM port\", \"Temp Delay Lps\", \"Temp Value\", \"Fail Loops\", \"Temp Test Cal\", \"Amps Fail level\", \"Mail Test File To:\", \"Mail Test Fail\": Value Change" {
                  selector: _ -> [_ _ _]
                  dyn-events: _ -> [_ _ _]
                  timeout: 10.0 -> [_ _ _]
                  tunnel: w5141 -> [_ w5143 _]
                  tunnel: w5140 -> [_ w5144 _]
                  tunnel: w5139 -> [_ _ w5155]
                  event Timeout {
                    n2813 = event-data() -> ()  [unwired: 1 in, 3 out]
                  }
                  event "SET LAB01-1", "SET LAB01-2", "SET LAB02-1", "SET LAB02-2", "SET LAB03-1", "SET LAB03-2", "SET LAB04-1", "SET LAB04-2", "SET LAB05-1", "SET LAB05-2", "Network Directory", "C drive data root dir", "RATE (Hz)", "SAMPLES", "Select COM port", "Temp Delay Lps", "Temp Value", "Fail Loops", "Temp Test Cal", "Amps Fail level", "Mail Test File To:", "Mail Test Fail": Value Change {
                    n2814 = event-data() -> ()  [unwired: 1 in, 6 out]
                    n2815 = Open/Create/Replace File(file path (use dialog)=w5143, operation (0:open)=T17."replace or create") -> (refnum out=w5149:refnum<file>, error out=w5148:errorcluster)  [unwired: 4 in, 1 out]
                    n2816 = Write to Binary File(file (use dialog)=w5149, data=w5144, error in=w5148) -> (refnum out=w5147:refnum<file>, error out=w5146:errorcluster)  [unwired: 3 in, 1 out]
                    n2817 = Close File(refnum=w5147, error in=w5146) -> (error out=w5145:errorcluster)  [unwired: 1 out]
                    n2818 = local write "data file error"(w5145) -> ()
                  }
                  event "MAIL SETTINGS.OUT SERVER ADDRESS", "MAIL SETTINGS.FROM ACCOUNT", "MAIL SETTINGS.USER NAME", "MAIL SETTINGS.PASSWORD", "Auto Mail Send", "TO (string):": Value Change {
                    n2819 = event-data() -> ()  [unwired: 1 in, 6 out]
                    n2820 = local read "MAIL SETTINGS"() -> (w5154:T7)
                    n2821 = local read "Auto Mail Send"() -> (w5152:bool)
                    n2822 = local read "TO (string):"() -> (w5151:string)
                    n2823 = Open/Create/Replace File(file path (use dialog)=w5155, operation (0:open)=T17."replace or create") -> (refnum out=w5160:refnum<file>, error out=w5159:errorcluster)  [unwired: 4 in, 1 out]
                    n2824 = Bundle("MAIL SETTINGS"=w5154, "Auto Mail Send"=w5152, "TO (string):"=w5151) -> (w5153:T43)  [unwired: 1 in]
                    n2825 = Write to Binary File(file (use dialog)=w5160, data=w5153, error in=w5159) -> (refnum out=w5158:refnum<file>, error out=w5157:errorcluster)  [unwired: 3 in, 1 out]
                    n2826 = Close File(refnum=w5158, error in=w5157) -> (error out=w5156:errorcluster)  [unwired: 1 out]
                    n2827 = local write "data file error"(w5156) -> ()
                  }
                }
              }
            }
          }
          frame #18 {
            # "mail control"
            n2828 = local read "MAIL SETTINGS"() -> (w5177:T7)
            n2829 = local read "Auto Mail Send"() -> (w5163:bool)
            n2830 = Unbundle(w5177) -> ("OUT SERVER ADDRESS"=w5176:string, "FROM ACCOUNT"=w5175:string, "TEST MAIL"=w5174:bool)  [unwired: 4 out]
            n2831 = stacked-sequence {
              tunnel: "TO (string):" -> [_ w5216]
              tunnel: w5177 -> [w5182 w5215]
              tunnel: w5176 -> [w5181 w5214]
              tunnel: w5175 -> [w5180 w5213]
              tunnel: w5174 -> [w5179 _]
              tunnel: w5163 -> [_ w5212]
              tunnel: w5173 -> [_ w5211]
              tunnel: w5172 -> [_ w5210]
              tunnel: w5171 -> [_ w5209]
              tunnel: w5170 -> [_ w5208]
              tunnel: w5169 -> [_ w5207]
              tunnel: w5168 -> [_ w5206]
              tunnel: w5167 -> [_ w5205]
              tunnel: w5166 -> [_ w5204]
              tunnel: w5165 -> [_ w5203]
              tunnel: w5164 -> [_ w5202]
              tunnel: "TO (string):" -> [w5178 _]
              frame #0 {
                # "mail test"
                n2832 = case shown="True" w5179 {
                  tunnel: w5182 -> [_ w5186]
                  tunnel: w5178 -> [_ w5185]
                  tunnel: w5181 -> [_ w5184]
                  tunnel: w5180 -> [_ w5183]
                  frame False {
                  }
                  frame True {
                    n2833 = stacked-sequence {
                      seq-local: [_ _ w5196 _] -> [_ _ _ w5197]
                      tunnel: w5186 -> [w5189 _ _ w5201]
                      tunnel: w5185 -> [_ _ w5194 _]
                      tunnel: w5184 -> [_ _ w5192 _]
                      tunnel: w5183 -> [_ _ w5193 _]
                      frame #0 {
                        n2834 = Bundle(cluster=w5189, "TEST MAIL STATUS"="TEST START") -> (w5187:T7)  [unwired: 6 in]
                        n2835 = local write "MAIL SETTINGS"(w5187) -> ()
                      }
                      frame #1 {
                        n2836 = Wait (ms)(milliseconds to wait=500) -> ()  [unwired: 1 out]
                      }
                      frame #2 {
                        n2837 = call "sub vi - send mail v5.vi"("TO:"=w5194, "subject"="MAIL TEST FROM LAB PANEL", "from"=w5193, "out going server"=w5192, "message"="TEST MESSAGE") -> ("error out"=w5196:errorcluster)  [unwired: 10 in]
                      }
                      frame #3 {
                        n2838 = Bundle(cluster=w5201, "TEST MAIL"=FALSE, "TEST MAIL STATUS"="TEST END", "mail error"=w5197) -> (w5199:T7)  [unwired: 4 in]
                        n2839 = local write "MAIL SETTINGS"(w5199) -> ()
                      }
                    }
                  }
                }
              }
              frame #1 {
                # "mail report"
                n2840 = stacked-sequence {
                  seq-local: [_ w5259 _ _] -> [_ _ _ w5449]
                  seq-local: [_ _ w5362 _] -> [_ _ _ w5439]
                  seq-local: [w5226 _ _ _] -> [_ w5276 _ _]
                  seq-local: [w5225 _ _ _] -> [_ w5275 _ _]
                  seq-local: [w5223 _ _ _] -> [_ w5273 _ _]
                  seq-local: [w5224 _ _ _] -> [_ w5274 _ _]
                  seq-local: [w5222 _ _ _] -> [_ w5272 _ _]
                  seq-local: [w5221 _ _ _] -> [_ w5267 _ _]
                  seq-local: [w5220 _ _ _] -> [_ w5268 _ _]
                  seq-local: [w5219 _ _ _] -> [_ w5269 _ _]
                  seq-local: [w5218 _ _ _] -> [_ w5270 _ _]
                  seq-local: [w5217 _ _ _] -> [_ w5271 _ _]
                  tunnel: w5216 -> [_ _ _ w5450]
                  tunnel: w5215 -> [_ _ _ w5433]
                  tunnel: w5214 -> [_ _ _ w5447]
                  tunnel: w5213 -> [_ _ _ w5446]
                  tunnel: w5212 -> [w5257 _ _ w5441]
                  tunnel: w5211 -> [_ _ w5392 _]
                  tunnel: w5210 -> [_ _ w5389 _]
                  tunnel: w5209 -> [_ _ w5388 _]
                  tunnel: w5208 -> [_ _ w5387 _]
                  tunnel: w5207 -> [_ _ w5386 _]
                  tunnel: w5206 -> [_ _ w5385 _]
                  tunnel: w5205 -> [_ _ w5384 _]
                  tunnel: w5204 -> [_ _ w5383 _]
                  tunnel: w5203 -> [_ _ w5382 _]
                  tunnel: w5202 -> [_ _ w5381 _]
                  frame #0 {
                    n2841 = case shown="False" w5257 {
                      frame False {
                        n2842 = local write "mail control"("") -> ()
                      }
                      frame True {
                      }
                    }
                    n2843 = local read "SET LAB01-1"() -> (w5256:T5)
                    n2844 = local read "SET LAB01-2"() -> (w5255:T5)
                    n2845 = local read "SET LAB02-1"() -> (w5254:T5)
                    n2846 = local read "SET LAB02-2"() -> (w5253:T5)
                    n2847 = local read "SET LAB03-1"() -> (w5252:T5)
                    n2848 = local read "SET LAB04-1"() -> (w5250:T5)
                    n2849 = local read "SET LAB05-1"() -> (w5248:T5)
                    n2850 = local read "SET LAB03-2"() -> (w5251:T5)
                    n2851 = local read "SET LAB04-2"() -> (w5249:T5)
                    n2852 = local read "SET LAB05-2"() -> (w5247:T5)
                    n2853 = Unbundle(w5252) -> ("DESCRIPTION"=w5232:string)  [unwired: 4 out]
                    n2854 = Unbundle(w5251) -> ("DESCRIPTION"=w5231:string)  [unwired: 4 out]
                    n2855 = Unbundle(w5250) -> ("DESCRIPTION"=w5230:string)  [unwired: 4 out]
                    n2856 = Unbundle(w5247) -> ("DESCRIPTION"=w5227:string)  [unwired: 4 out]
                    n2857 = Unbundle(w5253) -> ("DESCRIPTION"=w5233:string)  [unwired: 4 out]
                    n2858 = Unbundle(w5249) -> ("DESCRIPTION"=w5229:string)  [unwired: 4 out]
                    n2859 = Unbundle(w5256) -> ("DESCRIPTION"=w5245:string)  [unwired: 4 out]
                    n2860 = Unbundle(w5254) -> ("DESCRIPTION"=w5234:string)  [unwired: 4 out]
                    n2861 = Unbundle(w5248) -> ("DESCRIPTION"=w5228:string)  [unwired: 4 out]
                    n2862 = Unbundle(w5255) -> ("DESCRIPTION"=w5235:string)  [unwired: 4 out]
                    n2863 = Concatenate Strings("[LAB05-2/", w5227) -> (w5217:string)
                    n2864 = Concatenate Strings("[LAB05-1/", w5228) -> (w5218:string)
                    n2865 = Concatenate Strings("[LAB04-2/", w5229) -> (w5219:string)
                    n2866 = Concatenate Strings("[LAB03-2/", w5231) -> (w5221:string)
                    n2867 = Concatenate Strings("[LAB04-1/", w5230) -> (w5220:string)
                    n2868 = Concatenate Strings("[LAB03-1/", w5232) -> (w5222:string)
                    n2869 = Concatenate Strings("[LAB01-2/", w5235) -> (w5225:string)
                    n2870 = Concatenate Strings("[LAB02-2/", w5233) -> (w5223:string)
                    n2871 = Concatenate Strings("[LAB01-1/", w5245) -> (w5226:string)
                    n2872 = Concatenate Strings("[LAB02-1/", w5234) -> (w5224:string)
                  }
                  frame #1 {
                    w5280 = "/"
                    w5281 = 2.0
                    n2873 = local read "DISP LAB01-2"() -> (w5360:T4)
                    n2874 = local read "DISP LAB01-1"() -> (w5361:T4)
                    n2875 = local read "DISP LAB02-1"() -> (w5359:T4)
                    n2876 = local read "DISP LAB03-2"() -> (w5356:T4)
                    n2877 = local read "DISP LAB02-2"() -> (w5358:T4)
                    n2878 = local read "DISP LAB03-1"() -> (w5357:T4)
                    n2879 = local read "DISP LAB04-2"() -> (w5354:T4)
                    n2880 = local read "DISP LAB04-1"() -> (w5355:T4)
                    n2881 = local read "DISP LAB05-1"() -> (w5353:T4)
                    n2882 = local read "DISP LAB05-2"() -> (w5352:T4)
                    n2883 = Unbundle(w5360) -> ("CYCLE"=w5344:dbl, "MINS"=w5343:dbl, "STATUS"=w5340:string)
                    n2884 = Unbundle(w5361) -> ("CYCLE"=w5349:dbl, "MINS"=w5348:dbl, "STATUS"=w5345:string)
                    n2885 = Unbundle(w5359) -> ("CYCLE"=w5337:dbl, "MINS"=w5336:dbl, "STATUS"=w5335:string)
                    n2886 = Unbundle(w5356) -> ("CYCLE"=w5324:dbl, "MINS"=w5323:dbl, "STATUS"=w5320:string)
                    n2887 = Unbundle(w5357) -> ("CYCLE"=w5329:dbl, "MINS"=w5328:dbl, "STATUS"=w5325:string)
                    n2888 = Unbundle(w5358) -> ("CYCLE"=w5334:dbl, "MINS"=w5333:dbl, "STATUS"=w5330:string)
                    n2889 = Unbundle(w5355) -> ("CYCLE"=w5319:dbl, "MINS"=w5318:dbl, "STATUS"=w5315:string)
                    n2890 = Unbundle(w5354) -> ("CYCLE"=w5314:dbl, "MINS"=w5313:dbl, "STATUS"=w5310:string)
                    n2891 = Unbundle(w5353) -> ("CYCLE"=w5309:dbl, "MINS"=w5308:dbl, "STATUS"=w5305:string)
                    n2892 = Unbundle(w5352) -> ("CYCLE"=w5351:dbl, "MINS"=w5350:dbl, "STATUS"=w5302:string)
                    n2893 = Number To Decimal String(number=w5337) -> (decimal integer string=w5339:string)  [unwired: 1 in]
                    n2894 = Number To Decimal String(number=w5334) -> (decimal integer string=w5332:string)  [unwired: 1 in]
                    n2895 = Number To Decimal String(number=w5329) -> (decimal integer string=w5327:string)  [unwired: 1 in]
                    n2896 = Number To Decimal String(number=w5344) -> (decimal integer string=w5342:string)  [unwired: 1 in]
                    n2897 = Number To Decimal String(number=w5324) -> (decimal integer string=w5322:string)  [unwired: 1 in]
                    n2898 = Number To Decimal String(number=w5349) -> (decimal integer string=w5347:string)  [unwired: 1 in]
                    n2899 = Number To Decimal String(number=w5351) -> (decimal integer string=w5304:string)  [unwired: 1 in]
                    n2900 = Number To Decimal String(number=w5319) -> (decimal integer string=w5317:string)  [unwired: 1 in]
                    n2901 = Number To Decimal String(number=w5314) -> (decimal integer string=w5312:string)  [unwired: 1 in]
                    n2902 = Number To Decimal String(number=w5309) -> (decimal integer string=w5307:string)  [unwired: 1 in]
